vi "CLT_TriSpeedSP.vi"(8 "Empty in":dbl=8.5, 9 "Full in":dbl=2.0, 10 "Level PV":dbl, 11 "Level SP":dbl) -> (0 "OverDrain":bool=TRUE, 1 "OverFill":bool=TRUE, 2 "Pump Direction":enum16{"FILL", "DRAIN"}(ring), 3 "Pump Speed":enum16{"FAST", "SLOW", "CREEP", "STOP"}(ring))   [LabVIEW 2024]
doc: "The \"Run Test\" button selects between MANUAL adjustment of Set Point (SP) by the user or AUTO mode, where:\n1. Start, initial state drains until the tank is empty\n2. Filling, Auto set of SP to Max Fill Inches (or recipie)\n3. FULL Pause when full\n4. Draining Auto set of SP to 0 (or recipie)\n5. EMPTY Paue when empty\n6. Done SP set to 0."
panel:
  out "SP Out":dbl
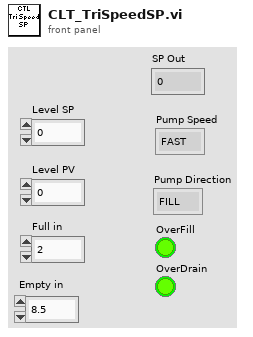
[diagram p1: front panel]
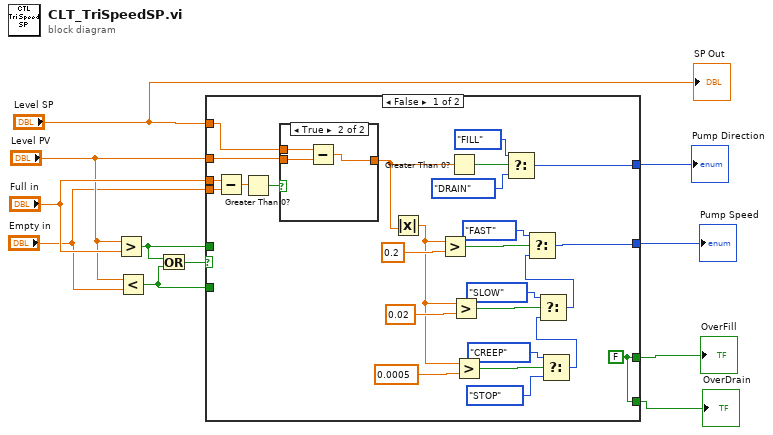
[diagram p0: block diagram]
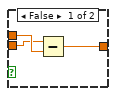
[diagram p2: hidden frame]
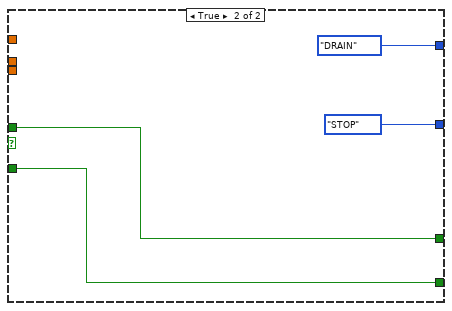
[diagram p3: hidden frame]
diagram:
  n1 = Greater?(x="Level PV", y="Full in") -> (0:w3:bool)
  n2 = Less?(x="Level PV", y="Empty in") -> (x < y?=w1:bool)
  n3 = Or(x=w3, y=w1) -> (x .or. y?=w5:bool)
  n4 = case shown="False" w5 {
    tunnel: "Level SP" -> [w13 _]
    tunnel: [w31 enum16{"FILL", "DRAIN"}."DRAIN" ("Pump Direction")] -> w10
    tunnel: [w18 enum16{"FAST", "SLOW", "CREEP", "STOP"}."STOP" ("Pump Speed")] -> w9
    tunnel: "Full in" -> [w17 _]
    tunnel: "Level PV" -> [w12 _]
    tunnel: "Empty in" -> [w16 _]
    tunnel: [w15 w45] -> w4
    tunnel: w3 -> [_ w45]
    tunnel: [w15 w44] -> w2
    tunnel: w1 -> [_ w44]
    frame False {
      w15 = FALSE
      n5 = Subtract(x=w17, y=w16) -> (x-y=w37:dbl)
      n6 = Greater Than 0?(x=w37) -> (x > 0?=w36:bool)
      n7 = case shown="True" w36 {
        tunnel: [w38 w43] -> w33
        tunnel: w13 -> [w40 w42]
        tunnel: w12 -> [w39 w41]
        frame False {
          n8 = Subtract(x=w39, y=w40) -> (x-y=w38:dbl)
        }
        frame True {
          n9 = Subtract(x=w42, y=w41) -> (x-y=w43:dbl)
        }
      }
      n10 = Absolute Value(x=w33) -> (abs(x)=w14:dbl)
      n11 = Greater?(x=w14, y=0.2) -> (0:w34:bool)
      n12 = Greater Than 0?(x=w33) -> (x > 0?=w32:bool)
      n13 = Greater?(x=w14, y=0.02) -> (0:w26:bool)
      n14 = Greater?(x=w14, y=0.0005) -> (0:w22:bool)
      n15 = Select(t=enum16{"FILL", "DRAIN"}."FILL" ("Pump Direction"), s=w32, f=enum16{"FILL", "DRAIN"}."DRAIN" ("Pump Direction")) -> (s? t:f=w31:enum16{"FILL", "DRAIN"})
      n16 = Select(t=enum16{"FAST", "SLOW", "CREEP", "STOP"}."CREEP" ("Pump Speed"), s=w22, f=enum16{"FAST", "SLOW", "CREEP", "STOP"}."STOP" ("Pump Speed")) -> (s? t:f=w19:enum16{"FAST", "SLOW", "CREEP", "STOP"})
      n17 = Select(t=enum16{"FAST", "SLOW", "CREEP", "STOP"}."SLOW" ("Pump Speed"), s=w26, f=w19) -> (s? t:f=w24:enum16{"FAST", "SLOW", "CREEP", "STOP"})
      n18 = Select(t=enum16{"FAST", "SLOW", "CREEP", "STOP"}."FAST" ("Pump Speed"), s=w34, f=w24) -> (s? t:f=w18:enum16{"FAST", "SLOW", "CREEP", "STOP"})
    }
    frame True {
    }
  }
  "Pump Speed" <- w9
  "Pump Direction" <- w10
  "OverFill" <- w4
  "OverDrain" <- w2
  "SP Out" <- "Level SP"
